vi "NameData_Array Names Build.vi"(8 "Error":errorcluster, 11 "Array Variant":variant) -> (0 "Error Out":errorcluster, 3 "Name Array Out":string[](array[string]))   [LabVIEW 2015]
uses:
  TypeDefs_Utility/ENUM_String_Between tolkens.ctl
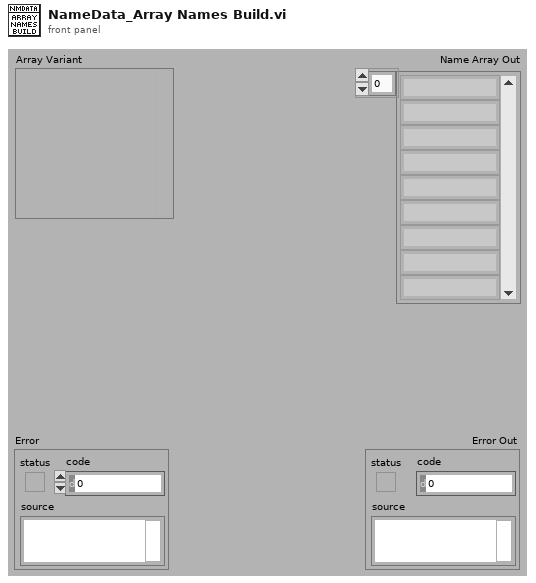
[diagram p1: front panel]
types:
  T1 = typedef "ENUM_String_Between tolkens.ctl" = enum16{"Braces;{}", "Brackets;[]", "Parens;()", "Angles;<>", "Colens;::", "Quotes;\"\"", "Backslashes;\\\\", "None;"}
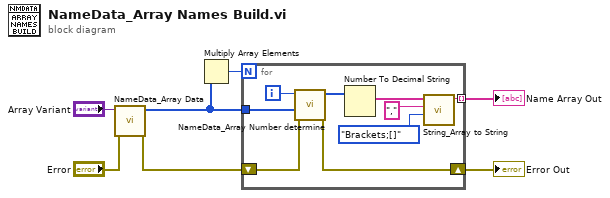
[diagram p0: block diagram]
diagram:
  n1 = call "NameData_Array Data.vi"("Error"="Error", "Array Variant"="Array Variant") -> ("Error Out"=w2:errorcluster, "Dim Sizes Out"=w5:u32[])  [unwired: 6 in, 2 out]
  n2 = Multiply Array Elements(1:w5) -> (0:w6:u32)
  n3 = for {
    N: w6 -> [_]
    tunnel: w5 -> [w11]
    tunnel: [w13] -> w7 mode=indexing
    shift-right: [w8] -> w1
    shift-left: w2 -> [w9]
    i -> [w16]
    n4 = call "NameData_Array Number determine.vi"("Error"=w9, "Dim Sizes"=w11, "Row Index"=w16) -> ("Error Out"=w8:errorcluster, "Row Numbers Out"=w10:u32[])  [unwired: 7 in]
    n5 = Number To Decimal String(number=w10) -> (decimal integer string=w15:string[])  [unwired: 1 in]
    n6 = call "String_Array to String.vi"("Surround Chars"=ENUM_String_Between_tolkens."Brackets;[]", "Seperator(,)"=",", "String Array"=w15) -> ("String Out"=w13:string)  [unwired: 8 in]
  }
  "Error Out" <- w1
  "Name Array Out" <- w7
